vi "Evaluate Part 2.vi"() -> ()   [LabVIEW 2021]
uses:
  Proto/Group.lvclass
panel:
  out "sum":u64
  in  "String":string="???.### 1,1,3\n.??..??...?##. 1,1,3\n?#?#?#?#?#?#?#? 1,3,1,6\n????.#...#... 4,1,1\n????.######..#####. 1,6,5\n?###???????? 3,2,1"
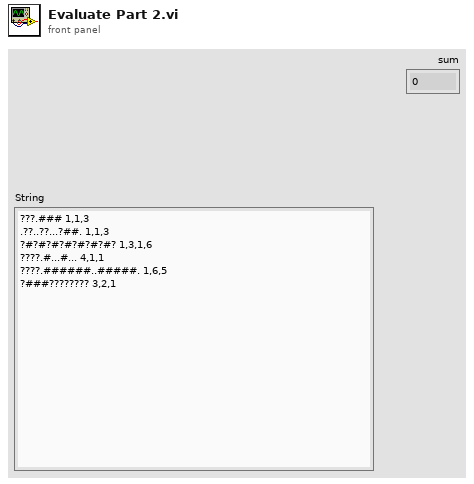
[diagram p1: front panel]
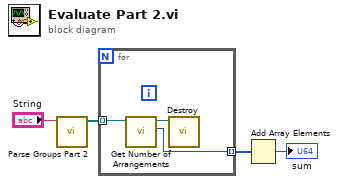
[diagram p0: block diagram]
diagram:
  n1 = call "Parse Groups Part 2.vi"("Input"="String") -> ("Groups"=w1:refnum<class "Group.lvclass">[])  [unwired: 10 in]
  n2 = for {
    tunnel: w1 -> [w6] mode=indexing
    tunnel: [w5] -> w3 mode=indexing
    n3 = call "Get Number of Arrangements.vi"("Proto in"=w6) -> ("Arrangements"=w5:u64, "Proto out"=w7:refnum<class "Group.lvclass">)  [unwired: 8 in, 1 out]
    n4 = call "Destroy.vi"("Group"=w7) -> ()  [unwired: 10 in, 1 out]
  }
  n5 = Add Array Elements(numeric array=w3) -> (sum=→"sum":u64)
